vi "init_drive.vi"(9 "Tolerance (m)":dbl, 10 "Drive Location":T1 {"North" format="%#_10f"; "East" format="%#_8f"}) -> (2 "Mission.lvclass":refnum<class "Mission.lvclass">)   [LabVIEW 2011, in "Mission.lvclass"]
uses:
  Mission.lvclass
  2 Typedefs/UTM Location.ctl
  Mission.lvclass/Mission.ctl
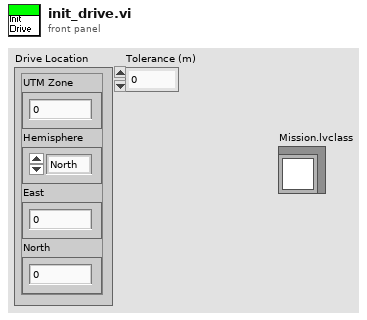
[diagram p1: front panel]
types:
  T1 = typedef "UTM Location.ctl" = cluster{"UTM Zone":dbl, "Hemisphere":enum16{"North", "South"}, "East":dbl, "North":dbl}
  T2 = enum16{"Round Buoy", "Drive", "Pass Buoys", "Station Keeping"}
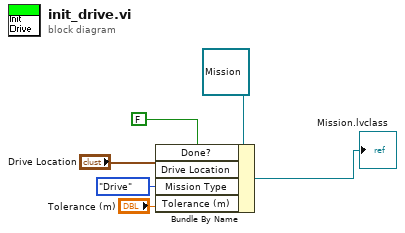
[diagram p0: block diagram]
diagram:
  n1 = Bundle By Name(cluster=refnum<class "Mission.lvclass"> refnum ("Mission Class"), "Done?"=FALSE, "Drive Location"="Drive Location", "Mission Type"=T2."Drive", "Tolerance (m)"="Tolerance (m)") -> (→"Mission.lvclass":refnum<class "Mission.lvclass">)
